vi "Get Builder Cluster.vi"(8 "error in (no error)":errorcluster, 9 "VI Refnum":refnum<vi>, 10 "Table Name":string, 11 "Panel Form Controller in":refnum<class "Panel Form Controller.lvclass">) -> (0 "error out":errorcluster, 2 "Builder Cluster":T1, 3 "Panel Form Controller out":refnum<class "Panel Form Controller.lvclass">)   [LabVIEW 2020, in "Panel Form Controller.lvlib" / "Panel Form Controller.lvclass"]
uses:
  Panel Form Controller.lvclass
  C:/Program Files (x86)/National Instruments/LabVIEW 2020/vi.lib/ActorFramework/Actor/Actor.lvclass
  Builder Cluster.ctl
  Database OOP/Table Libraries/Basic Form/Basic Form.lvclass
  Open Form Button/Open Form Button.lvclass
  <vilib>/ActorFramework/Actor/Actor.lvclass/Actor.ctl
  Panel Form Controller.lvclass/Panel Form Controller.ctl
  Configuration/Controller Configuration/Panel Form Controller Configuration.lvclass
  Panel Form Controller.lvlib
  <vilib>/ActorFramework/Actor/Actor.lvclass
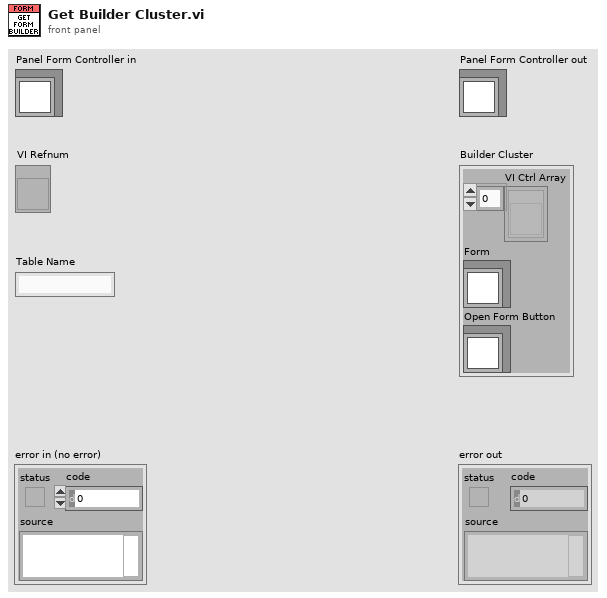
[diagram p1: front panel]
types:
  T1 = typedef "Panel Form Controller.lvlib/Builder Cluster.ctl" = cluster{"VI Ctrl Array":refnum<vi>[], "Form":refnum<class "Basic Form.lvclass">, "Open Form Button":refnum<class "Open Form Button.lvclass">}
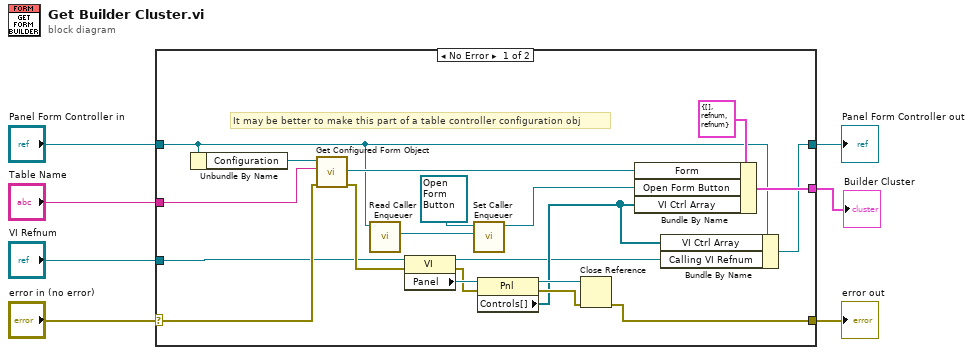
[diagram p0: block diagram]
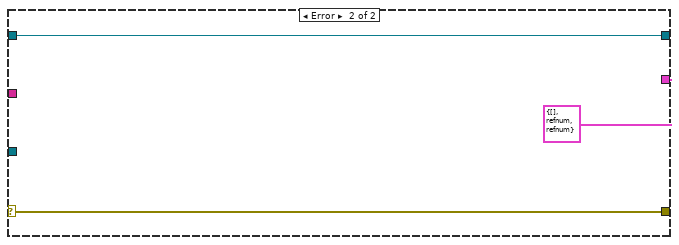
[diagram p2: hidden frame]
diagram:
  n1 = case shown="No Error" "error in (no error)" {
    selector: "error in (no error)" -> [w14 w30]
    tunnel: [w18 w30] -> w6
    tunnel: [w21 w29] -> w1
    tunnel: "Panel Form Controller in" -> [w10 w29]
    tunnel: "VI Refnum" -> [w8 _]
    tunnel: [w22 T1 {"VI Ctrl Array"=[], "Form"=refnum, "Open Form Button"=refnum} ("Builder Cluster")] -> w3
    tunnel: "Table Name" -> [w9 _]
    frame No Error {
      # "It may be better to make this part of a table controller configuration obj"
      n2 = Unbundle By Name(w10) -> ("Configuration"=w12:refnum<class "Panel Form Controller Configuration.lvclass">)
      n3 = call-dynamic "Get Configured Form Object.vi"("error in (no error)"=w14, "Table Name"=w9, "Panel Form Controller Configuration in"=w12) -> ("error out"=w13:errorcluster, "Configured Form"=w11:refnum<class "Basic Form.lvclass">)  [unwired: 6 in, 1 out]
      n4 = call <vilib>:"Read Caller Enqueuer.vi"("Actor"=w10) -> ("Caller Enqueuer"=w16:refnum<class "Message Enqueuer.lvclass">)  [unwired: 10 in]
      n5 = property class="VI"(reference=w8, error in=w13) -> (reference out=w19:refnum<vi>, error out=w26:errorcluster, "Panel"=w27:refnum<vi>)
      n6 = call "Set Caller Enqueuer.vi"("Caller Enqueuer"=w16, "Open Form Button in"=refnum<class "Open Form Button.lvclass"> refnum ("Panel Form Controller.lvlib:Open Form Button.lvclass")) -> ("Open Form Button out"=w15:refnum<class "Open Form Button.lvclass">)  [unwired: 8 in, 1 out]
      n7 = property class="Pnl"(reference=w27, error in=w26) -> (reference out=w24:refnum<vi>, error out=w23:errorcluster, "Controls[]"=w20:refnum<vi>[])
      n8 = Close Reference(reference=w24, error in (no error)=w23) -> (error out=w18:errorcluster)
      n9 = Bundle By Name(cluster=T1 {"VI Ctrl Array"=[], "Form"=refnum, "Open Form Button"=refnum} ("Builder Cluster"), "Form"=w11, "Open Form Button"=w15, "VI Ctrl Array"=w20) -> (w22:T1)
      n10 = Bundle By Name(cluster=w10, "VI Ctrl Array"=w20, "Calling VI Refnum"=w19) -> (w21:refnum<class "Panel Form Controller.lvclass">)
    }
    frame Error {
    }
  }
  "error out" <- w6
  "Panel Form Controller out" <- w1
  "Builder Cluster" <- w3
